vi "DAQ_main.vi"   [LabVIEW 2015]
uses:
  CONTROLS/Q_main_element.ctl
  CONTROLS/Q_DAQ_element.ctl
  <vilib>/DAQmx/write.llb/DAQmx Write (Digital Bool 1Line 1Point).vi
  <vilib>/DAQmx/read.llb/DAQmx Read (Digital Bool 1Line 1Point).vi
  <vilib>/DAQmx/read.llb/DAQmx Read (Counter U32 1Chan 1Samp).vi
  GLOBAL/Global_DAQ.vi
  GLOBAL/Global_ABORT.vi
  GLOBAL/Global_MAIN.vi
  <vilib>/DAQmx/create/channels.llb/DAQmx Create Channel (DO-Digital Output).vi
  <vilib>/DAQmx/miscellaneous.llb/DAQmx Fill In Error Info.vi
  <vilib>/DAQmx/create/channels.llb/DAQmx Create Channel (DI-Digital Input).vi
  <vilib>/DAQmx/create/channels.llb/DAQmx Create Channel (CI-Count Edges).vi
types:
  T1 = cluster{"Analogic input":tag, "size(s)":i32, " waveform":waveform(dbl)}[]
  T2 = cluster{"AOTF trigger task":refnum<k21>, "counter task":refnum<k21>}
  T3 = typedef "Q_DAQ_element.ctl" = cluster{"variant":variant, "Instruction":enum16{"DAQ_idle", "DAQ_initialize", "DAQ_error", "DAQ_security_stop", "DAQ_init_single_scan", "DAQ_single_scan", "DAQ_init_merFISH", "DAQ_scan_merFISH", "DAQ_photobleaching_merFISH", "DAQ_close_merFISH", "DAQ_stop"}}
  T4 = typedef "Q_main_element.ctl" = cluster{"variant":variant, "Instruction":enum16{"Main_idle", "Main_initialize", "Main_initialize_TDMS", "Main_initialize_Queue", "Main_error", "Main_DAQ_initialization_results", "Main_ASI_initialization_results", "Main_Piezo_initialization_results", "Main_Valve_initialization_results", "Main_Pump_initialization_results", "Main_CAMERA_initialization_results", "Main_FPGA_initialization_results", "Main_DAQ_error", "Main_ASI_error", "Main_Piezo_error", "Main_CAMERA_error", "Main_Valve_error", "Main_Pump_error", "Main_FPGA_error", "Main_start_acquiring", "Main_not_acquiring", "Main_acquiring", "Main_stop_acquiring", "Main_change_exposure", "Main_change_z_scan_parameters", "Main_define_ROI", "Main_define_mosaic", "Main_read_kinetic_time", "Main_cooler", "Main_read_temperature", "Main_save_XY", "Main_load_XY", "Main_discard_XY", "Main_move_to_XY", "Main_measure_QPD", "Main_autofocus_calibration", "Main_autofocus_initialization", "Main_autofocus_stop", "Main_save_PID", "Main_change_H_valve_position", "Main_two_way_valve", "Main_save_movie", "Main_init_single_scan", "Main_single_scan", "Main_stop_single_scan", "Main_merFISH_illumination_parameters", "Main_merFISH_buffer_probe_list", "Main_merFISH_injections_procedure", "Main_merFISH_save_setpoint", "Main_merFISH_DAPI_parameters", "Main_merFISH_Brightfield_parameters", "Main_merFISH_save_embryo_ROI", "Main_merFISH_init", "Main_merFISH_resume", "Main_merFISH_start_autofocus", "Main_merFISH_open_close_valve_merFISH", "Main_merFISH_open_close_valve_photobleaching", "Main_merFISH_hybridization", "Main_merFISH_move_to_ROI", "Main_merFISH_wait_stabilization", "Main_merFISH_move_to_REF", "Main_merFISH_scan", "Main_merFISH_photobleaching_injection", "Main_merFISH_photobleaching", "Main_merFISH_send_email", "Main_merFISH_close", "Main_STOP"}}
  T5 = enum16{"DAQ_idle", "DAQ_initialize", "DAQ_error", "DAQ_security_stop", "DAQ_init_single_scan", "DAQ_single_scan", "DAQ_init_merFISH", "DAQ_scan_merFISH", "DAQ_photobleaching_merFISH", "DAQ_close_merFISH", "DAQ_stop"}
  T6 = cluster{"Analogic input":tag, "size(s)":i32, " waveform":waveform(dbl)}
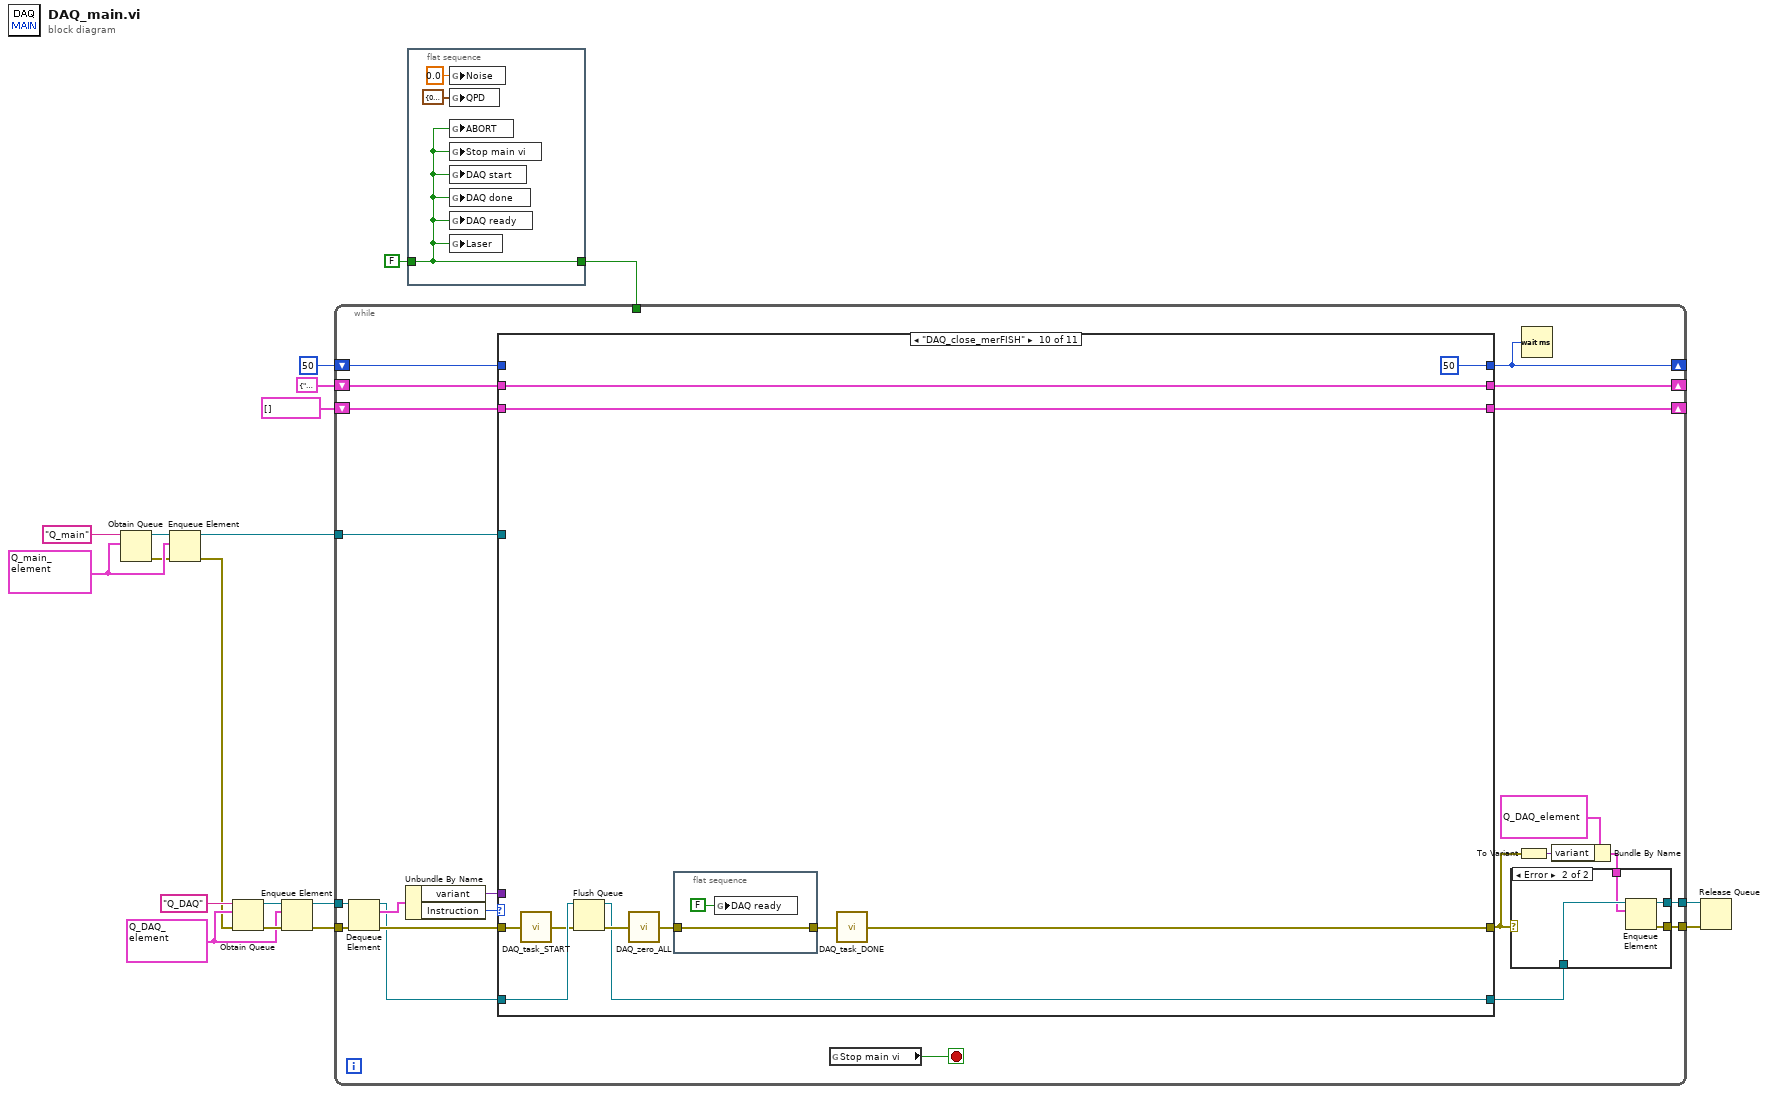
[diagram p0: block diagram]
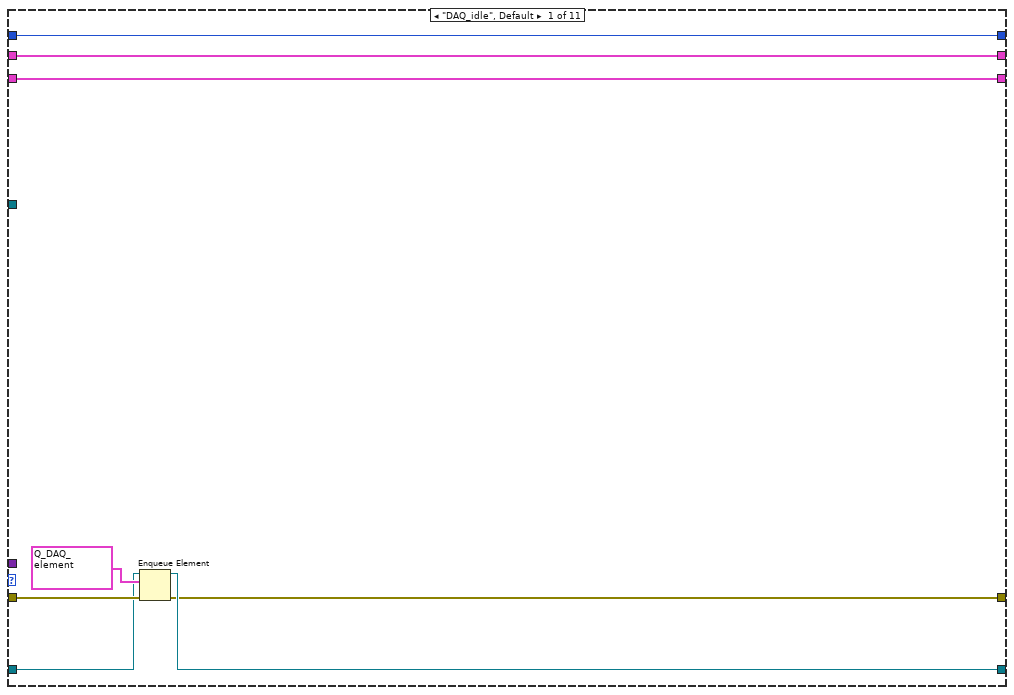
[diagram p3: hidden frame]
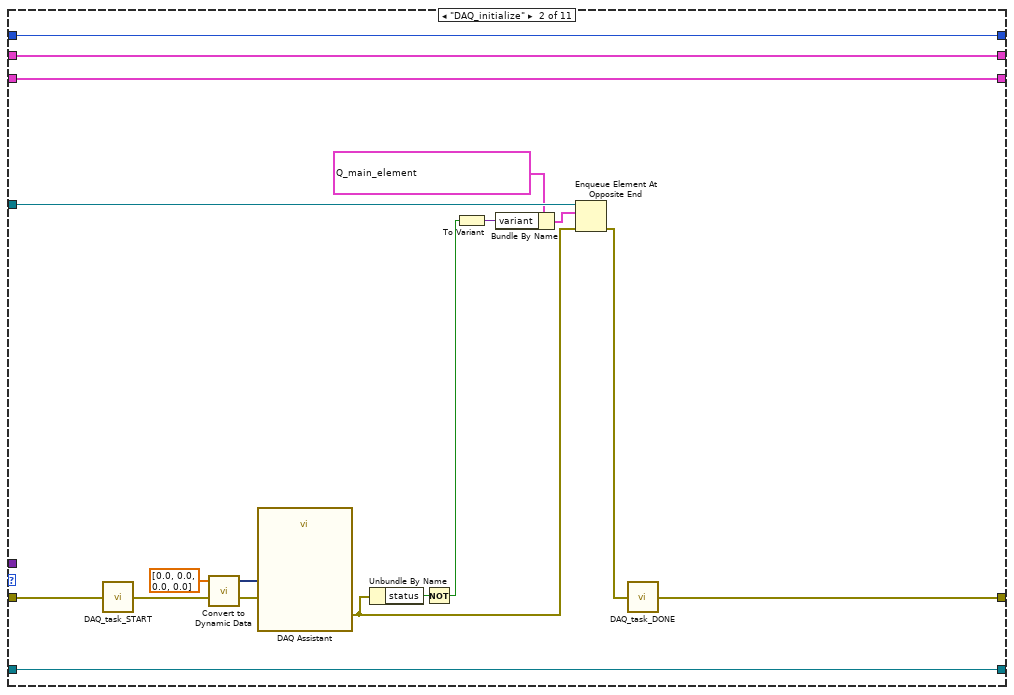
[diagram p4: hidden frame]
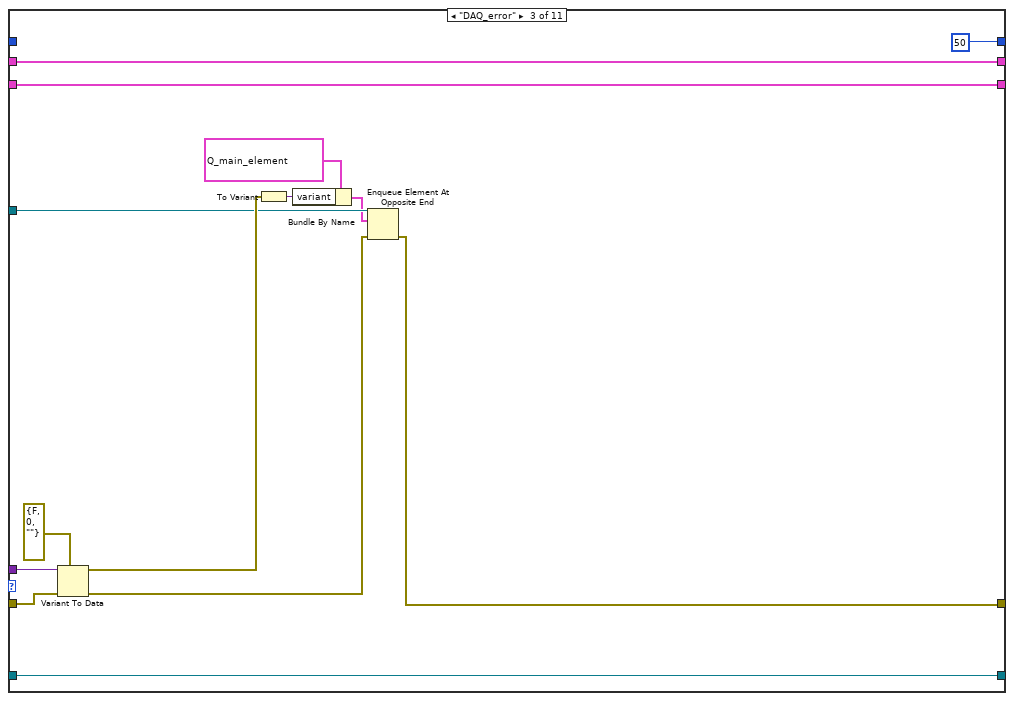
[diagram p5: hidden frame]
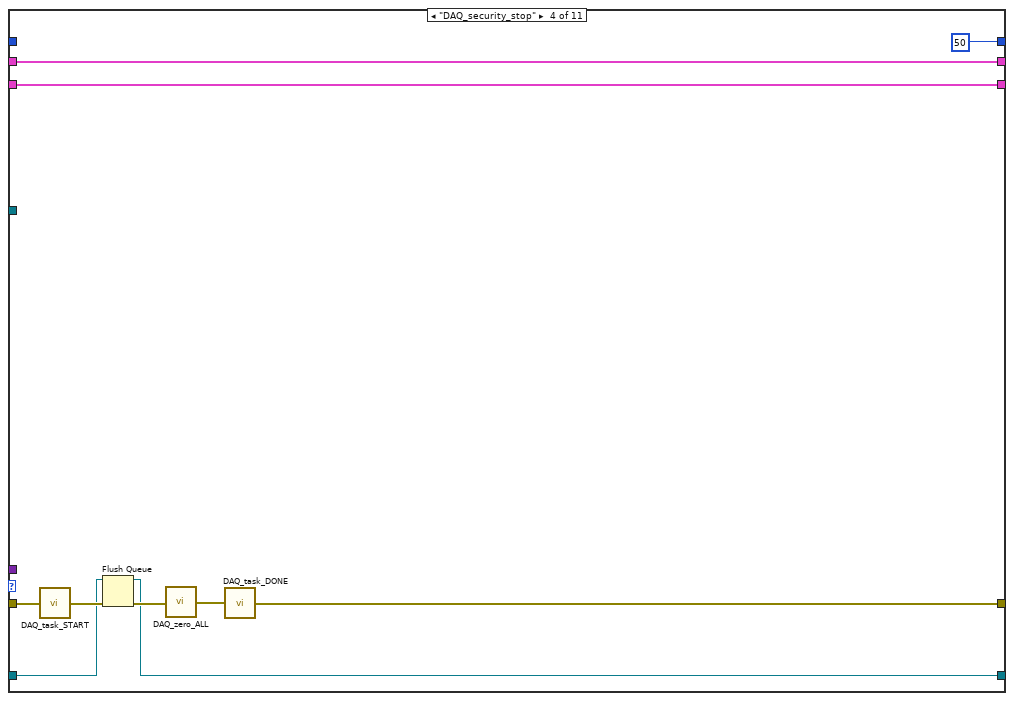
[diagram p6: hidden frame]
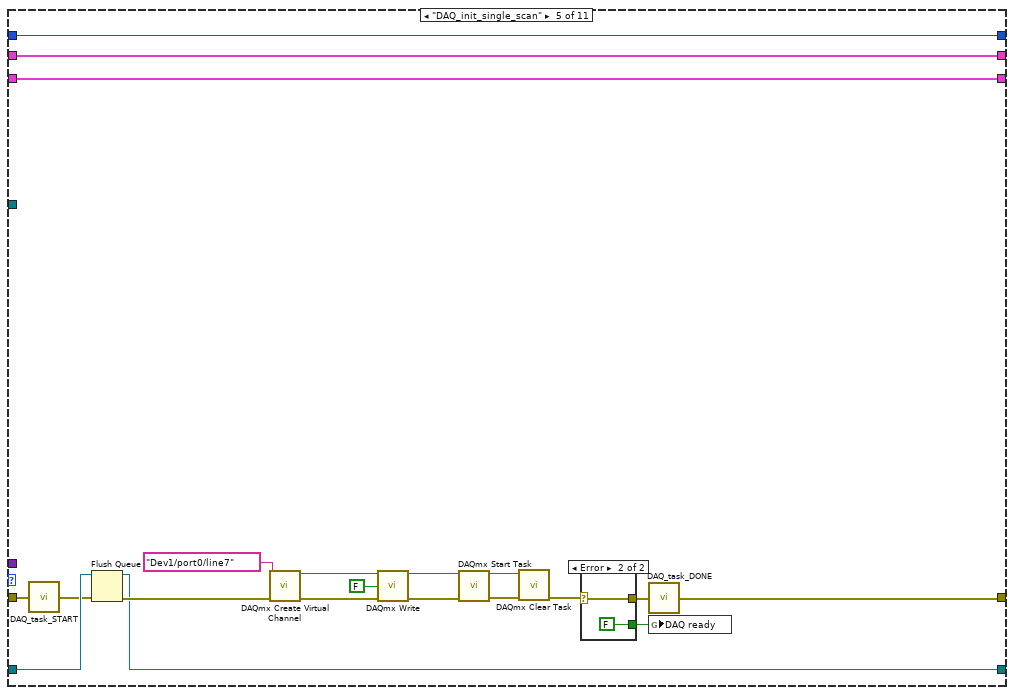
[diagram p7: hidden frame]
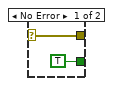
[diagram p8: hidden frame]
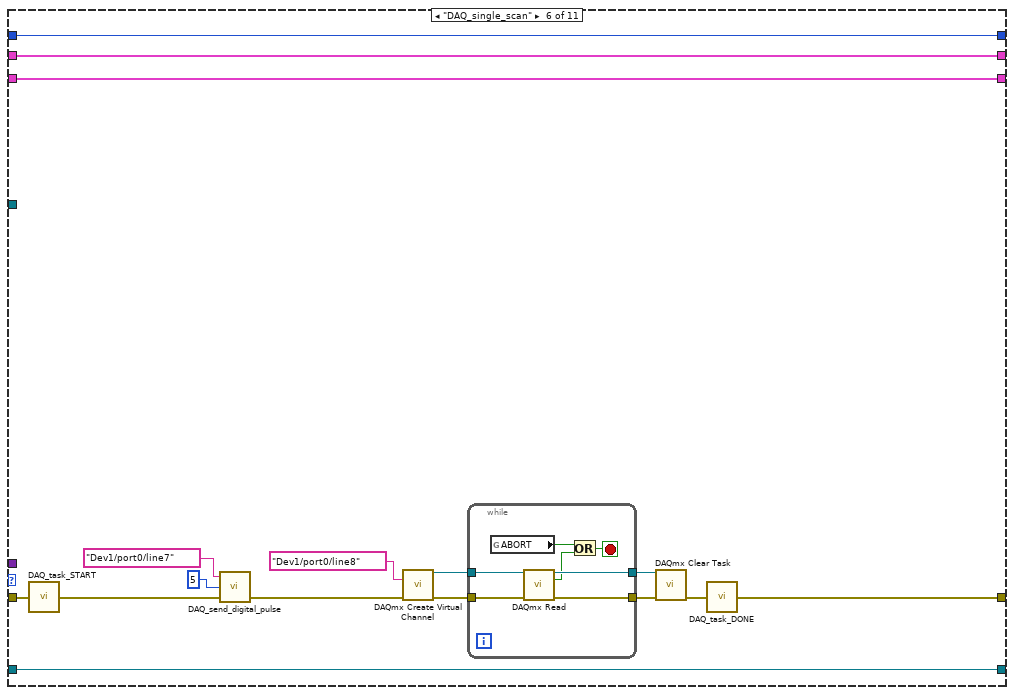
[diagram p9: hidden frame]
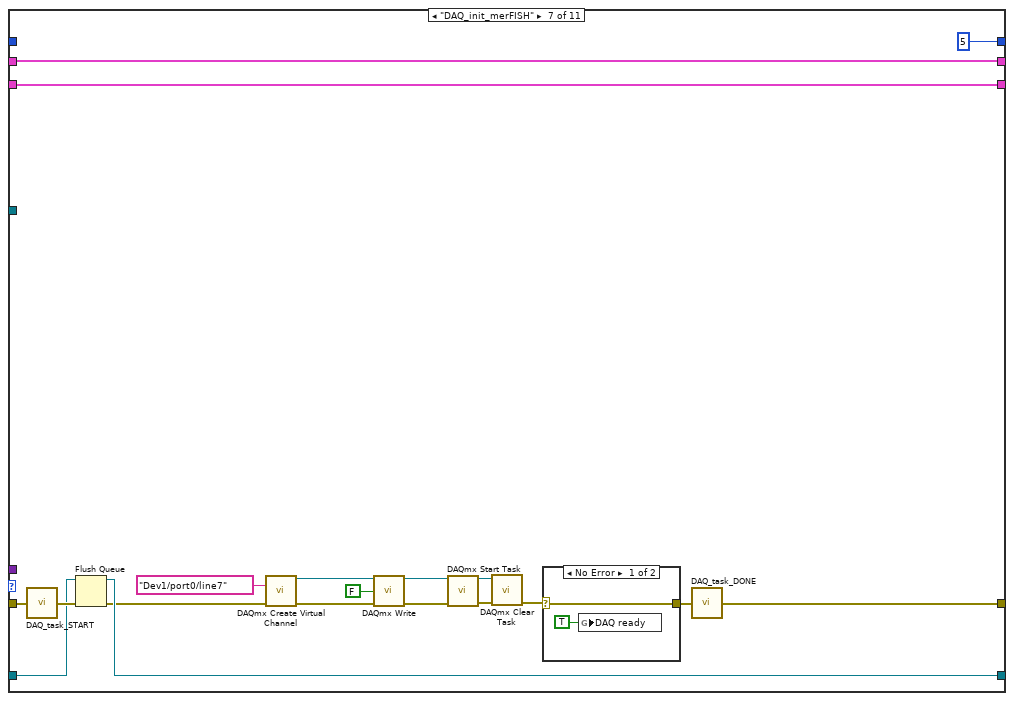
[diagram p10: hidden frame]
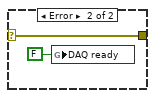
[diagram p11: hidden frame]
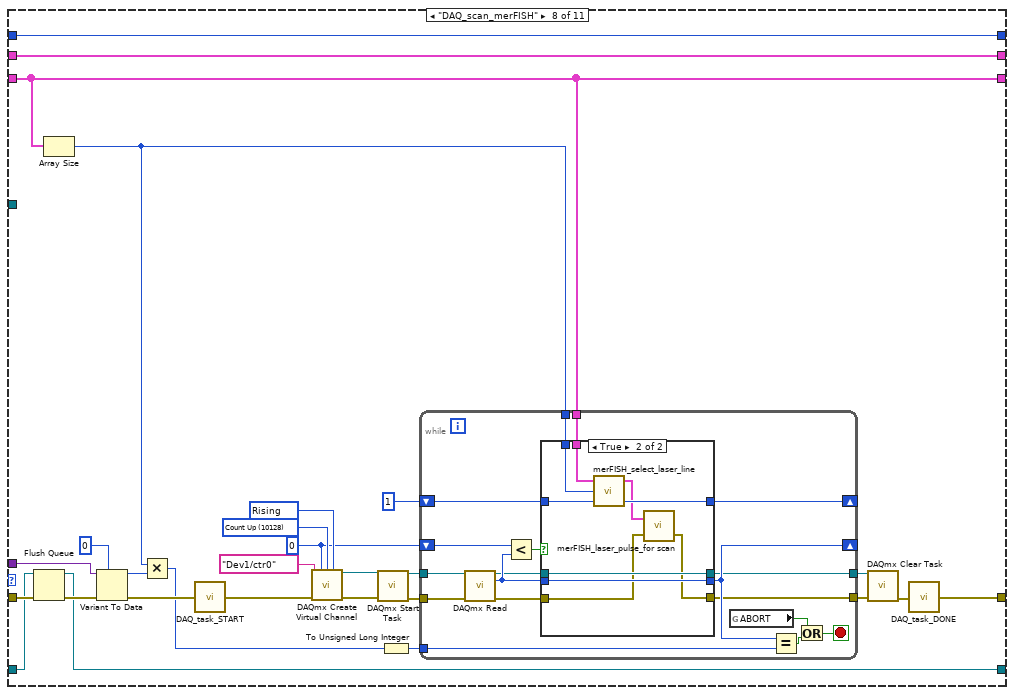
[diagram p12: hidden frame]
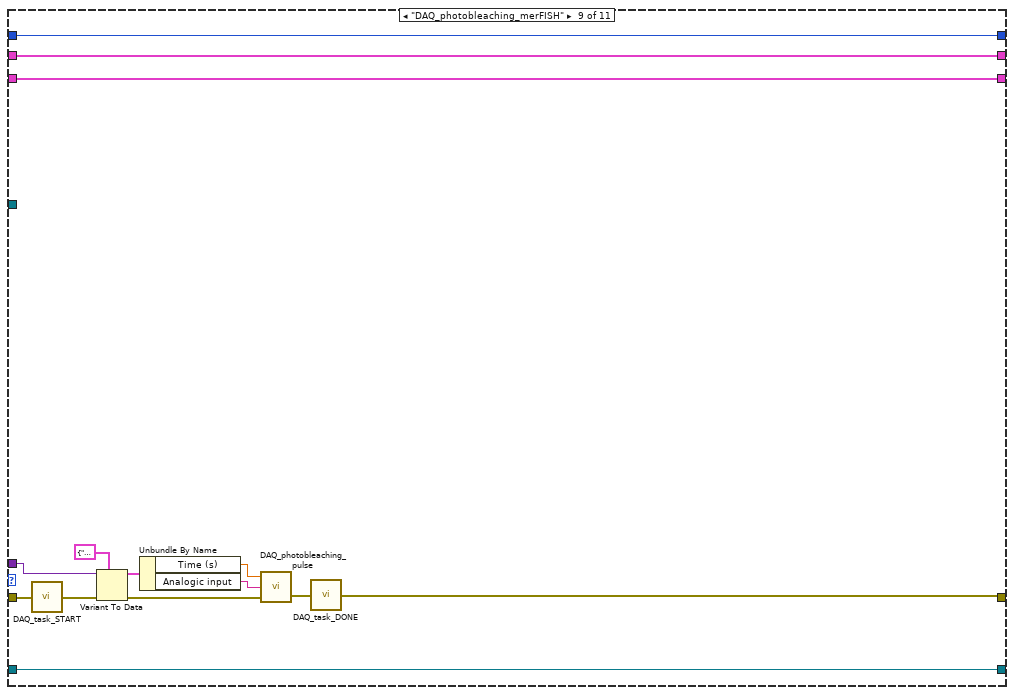
[diagram p14: hidden frame]
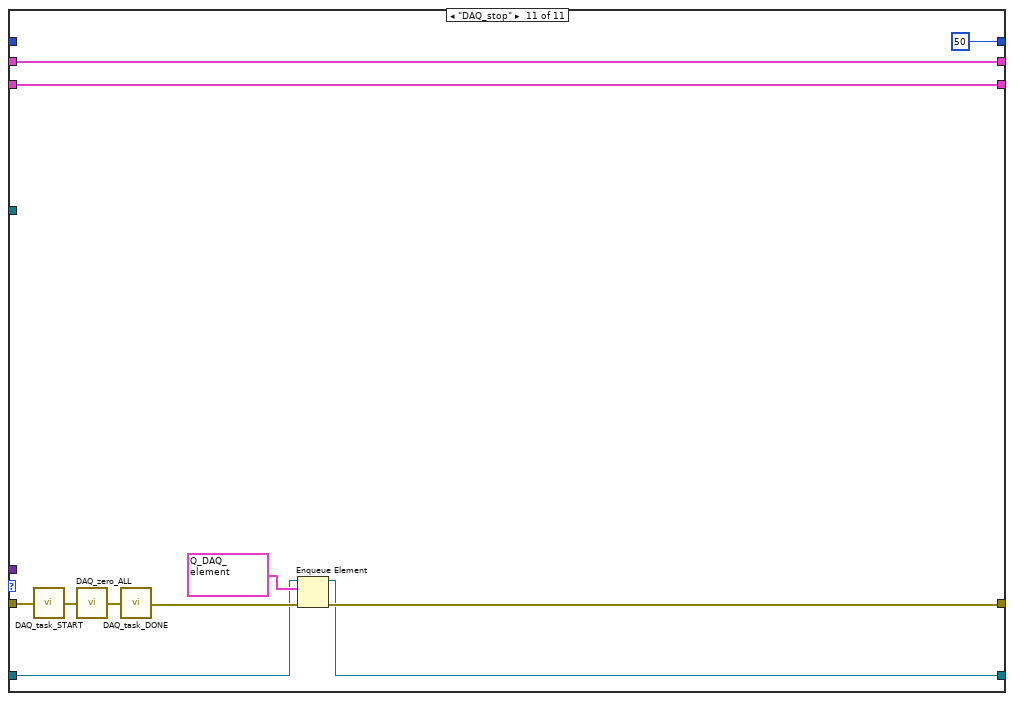
[diagram p15: hidden frame]
diagram:
  w5 = T3 {"variant"=variant, "Instruction"=enum."DAQ_idle"} ("Q_DAQ")
  w12 = T4 {"variant"=variant, "Instruction"=enum."Main_idle"} ("Q_main_element")
  n1 = Obtain Queue(name (unnamed)="Q_main", element data type=w12) -> (queue out=w10:refnum<queue>, error out=w11:errorcluster)  [unwired: 3 in, 1 out]
  n2 = Enqueue Element(queue=w10, element=w12, error in (no error)=w11) -> (queue out=w8:refnum<queue>, error out=w4:errorcluster)  [unwired: 1 in, 1 out]
  n3 = Obtain Queue(name (unnamed)="Q_DAQ", element data type=w5, error in (no error)=w4) -> (queue out=w18:refnum<queue>, error out=w17:errorcluster)  [unwired: 2 in, 1 out]
  n4 = Enqueue Element(queue=w18, element=w5, error in (no error)=w17) -> (queue out=w16:refnum<queue>, error out=w15:errorcluster)  [unwired: 1 in, 1 out]
  n5 = while {
    tunnel: w16 -> [w40]
    tunnel: w15 -> [w39]
    tunnel: [w36] -> w14
    tunnel: [w35] -> w13
    tunnel: w8 -> [w34]
    tunnel: w6 -> [_]
    shift-right: [w27] -> _
    shift-left: T2 {"AOTF trigger task"="", "counter task"=""} ("output cluster") -> [w28]
    shift-right: [w24] -> _
    shift-left: u32 50 ("milliseconds to wait") -> [w25]
    shift-right: [w23] -> _
    shift-left: T1 [] -> [w22]
    stop <- w41 stop-if-true
    n6 = Dequeue Element(queue=w40, error in (no error)=w39) -> (queue out=w21:refnum<queue>, element=w38:T3, error out=w37:errorcluster)  [unwired: 1 in, 1 out]
    n7 = Unbundle By Name(w38) -> ("variant"=w33:variant, "Instruction"=w26:T5)
    n8 = case shown="\"DAQ_close_merFISH\"" w26 {
      tunnel: w37 -> [w52 w57 w85 w96 w99 w133 w158 w192 w237 w245 w262]
      tunnel: [w48 w61 w76 w93 w97 w132 w162 w171 w239 w242 w256] -> w29
      tunnel: w34 -> [_ w70 w80 _ _ _ _ _ _ _ _]
      tunnel: w33 -> [_ _ w86 _ _ _ _ w177 w236 _ _]
      tunnel: w21 -> [w50 w58 w73 w94 w101 w131 w156 w191 w226 w248 w255]
      tunnel: w28 -> [w55 w63 w77 w92 w116 w136 w161 w193 w238 w250 w263]
      tunnel: [w55 w63 w77 w92 w116 w136 w161 w193 w238 w250 w263] -> w27
      tunnel: w25 -> [w54 w60 _ _ w115 w135 _ w194 w228 _ _]
      tunnel: [w54 w60 u32 50 ("milliseconds to wait") u32 50 ("milliseconds to wait") w115 w135 u32 5 ("milliseconds to wait") w194 w228 u32 50 ("milliseconds to wait") u32 50 ("milliseconds to wait")] -> w24
      tunnel: [w53 w59 w74 w88 w114 w134 w144 w181 w227 w246 w259] -> w23
      tunnel: w22 -> [w53 w59 w74 w88 w114 w134 w144 w181 w227 w246 w259]
      tunnel: [w49 w58 w73 w87 w100 w131 w155 w167 w226 w241 w254] -> w20
      frame "DAQ_idle", Default {
        n9 = Enqueue Element(queue=w50, element=T3 {"variant"=variant, "Instruction"=enum."DAQ_idle"} ("Q_DAQ"), error in (no error)=w52) -> (queue out=w49:refnum<queue>, error out=w48:errorcluster)  [unwired: 1 in, 1 out]
      }
      frame "DAQ_initialize" {
        n10 = call "DAQ_task_START.vi"("error in"=w57) -> ("error out"=w64:errorcluster)  [unwired: 1 in]
        n11 = call "Convert to Dynamic Data"("Array"=dbl[] [0.0, 0.0, 0.0, 0.0]) -> ("Dynamic Data Type"=w72:dynamicdata)  [unwired: 3 in]
        n12 = call "DAQ Assistant"("data"=w72, "error in"=w64) -> ("error out"=w62:errorcluster)  [unwired: 16 in, 1 out]
        n13 = Unbundle By Name(w62) -> ("status"=w66:bool)
        n14 = Not(x=w66) -> (.not. x?=w65:bool)
        n15 = To Variant(anything=w65) -> (Variant=w68:variant)
        n16 = Bundle By Name(cluster=T4 {"variant"=variant, "Instruction"=enum."Main_DAQ_initialization_results"} ("element"), "variant"=w68) -> (w67:T4)
        n17 = Enqueue Element At Opposite End(queue=w70, element=w67, error in (no error)=w62) -> (error out=w56:errorcluster)  [unwired: 1 in, 2 out]
        n18 = call "DAQ_task_DONE.vi"("error in"=w56) -> ("error out"=w61:errorcluster)
      }
      frame "DAQ_error" {
        n19 = Variant To Data(error in=w85, type=errorcluster {"status"=FALSE, "code"=0, "source"=""} ("error out"), Variant=w86) -> (data=w81:errorcluster, error out=w79:errorcluster)
        n20 = To Variant(anything=w81) -> (Variant=w82:variant)
        n21 = Bundle By Name(cluster=T4 {"variant"=variant, "Instruction"=enum."Main_DAQ_error"} ("Q_main_element"), "variant"=w82) -> (w78:T4)
        n22 = Enqueue Element At Opposite End(queue=w80, element=w78, error in (no error)=w79) -> (error out=w76:errorcluster)  [unwired: 1 in, 2 out]
      }
      frame "DAQ_security_stop" {
        n23 = call "DAQ_task_START.vi"("error in"=w96) -> ("error out"=w95:errorcluster)  [unwired: 1 in]
        n24 = Flush Queue(queue=w94, error in (no error)=w95) -> (queue out=w87:refnum<queue>, error out=w91:errorcluster)  [unwired: 1 out]
        n25 = call "DAQ_zero_ALL.vi"("error in"=w91) -> ("error out"=w90:errorcluster)
        n26 = call "DAQ_task_DONE.vi"("error in"=w90) -> ("error out"=w93:errorcluster)
      }
      frame "DAQ_init_single_scan" {
        n27 = call "DAQ_task_START.vi"("error in"=w99) -> ("error out"=w98:errorcluster)  [unwired: 1 in]
        n28 = Flush Queue(queue=w101, error in (no error)=w98) -> (queue out=w100:refnum<queue>, error out=w104:errorcluster)  [unwired: 1 out]
        n29 = call-poly <vilib>:"DAQmx Create Virtual Channel.vi"("lines"=tag "Dev1/port0/line7", "error in"=w104) -> ("task out"=w106:refnum<k21>, "error out"=w107:errorcluster)  [unwired: 12 in]
        n30 = call-poly <vilib>:"DAQmx Write.vi"("task/channels in"=w106, "data"=FALSE, "error in"=w107) -> ("task out"=w109:refnum<k21>, "error out"=w110:errorcluster)  [unwired: 10 in, 1 out]
        n31 = call <vilib>:"DAQmx Start Task.vi"("task/channels in"=w109, "error in"=w110) -> ("task out"=w111:refnum<k21>, "error out"=w112:errorcluster)  [unwired: 12 in]
        n32 = call <vilib>:"DAQmx Clear Task.vi"("task in"=w111, "error in"=w112) -> ("error out"=w113:errorcluster)  [unwired: 13 in]
        n33 = case shown="Error" w113 {
          selector: w113 -> [w118 w120]
          tunnel: [w118 w120] -> w102
          tunnel: [TRUE ("DAQ ready") FALSE ("DAQ ready")] -> w103
          frame No Error {
          }
          frame Error {
          }
        }
        n34 = call "DAQ_task_DONE.vi"("error in"=w102) -> ("error out"=w97:errorcluster)
        n35 = global write "Global_DAQ.vi" "DAQ ready"(w103) -> ()
      }
      frame "DAQ_single_scan" {
        n36 = call "DAQ_task_START.vi"("error in"=w133) -> ("error out"=w122:errorcluster)  [unwired: 1 in]
        n37 = call "DAQ_send_digital_pulse.vi"("error in"=w122, "Pulse length (ms)"=u32 5, "Digital input"=tag "Dev1/port0/line7") -> ("error out"=w125:errorcluster)  [unwired: 2 in]
        n38 = call-poly <vilib>:"DAQmx Create Virtual Channel.vi"("lines"=tag "Dev1/port0/line8", "error in"=w125) -> ("task out"=w128:refnum<k21>, "error out"=w127:errorcluster)  [unwired: 12 in]
        n39 = while {
          tunnel: w127 -> [w143]
          tunnel: w128 -> [w142]
          tunnel: [w141] -> w129
          tunnel: [w140] -> w130
          stop <- w139 stop-if-true
          n40 = global read "Global_ABORT.vi" "ABORT"() -> (w137:bool)
          n41 = call-poly <vilib>:"DAQmx Read.vi"("task/channels in"=w142, "error in"=w143) -> ("task out"=w141:refnum<k21>, "data"=w138:bool, "error out"=w140:errorcluster)  [unwired: 11 in]
          n42 = Or(x=w137, y=w138) -> (x .or. y?=w139:bool)
        }
        n43 = call <vilib>:"DAQmx Clear Task.vi"("task in"=w129, "error in"=w130) -> ("error out"=w121:errorcluster)  [unwired: 13 in]
        n44 = call "DAQ_task_DONE.vi"("error in"=w121) -> ("error out"=w132:errorcluster)
      }
      frame "DAQ_init_merFISH" {
        n45 = call "DAQ_task_START.vi"("error in"=w158) -> ("error out"=w157:errorcluster)  [unwired: 1 in]
        n46 = Flush Queue(queue=w156, error in (no error)=w157) -> (queue out=w155:refnum<queue>, error out=w146:errorcluster)  [unwired: 1 out]
        n47 = call-poly <vilib>:"DAQmx Create Virtual Channel.vi"("lines"=tag "Dev1/port0/line7", "error in"=w146) -> ("task out"=w148:refnum<k21>, "error out"=w149:errorcluster)  [unwired: 12 in]
        n48 = call-poly <vilib>:"DAQmx Write.vi"("task/channels in"=w148, "data"=FALSE, "error in"=w149) -> ("task out"=w151:refnum<k21>, "error out"=w152:errorcluster)  [unwired: 10 in, 1 out]
        n49 = call <vilib>:"DAQmx Start Task.vi"("task/channels in"=w151, "error in"=w152) -> ("task out"=w153:refnum<k21>, "error out"=w154:errorcluster)  [unwired: 12 in]
        n50 = call <vilib>:"DAQmx Clear Task.vi"("task in"=w153, "error in"=w154) -> ("error out"=w145:errorcluster)  [unwired: 13 in]
        n51 = case shown="No Error" w145 {
          selector: w145 -> [w164 w166]
          tunnel: [w164 w166] -> w160
          frame No Error {
            n52 = global write "Global_DAQ.vi" "DAQ ready"(TRUE ("DAQ ready")) -> ()
          }
          frame Error {
            n53 = global write "Global_DAQ.vi" "DAQ ready"(FALSE ("DAQ ready")) -> ()
          }
        }
        n54 = call "DAQ_task_DONE.vi"("error in"=w160) -> ("error out"=w162:errorcluster)
      }
      frame "DAQ_scan_merFISH" {
        w188 = 10280 items=["Rising"=10280, "Falling"=10171] ("edge")
        w189 = 10128 items=["Count Up"=10128, "Count Down"=10124, "Externally Controlled"=10326] ("count direction")
        w182 = u32 0 ("initial count")
        n55 = Flush Queue(queue=w191, error in (no error)=w192) -> (queue out=w167:refnum<queue>, error out=w179:errorcluster)  [unwired: 1 out]
        n56 = Array Size(array=w181) -> (size(s)=w174:i32)
        n57 = Variant To Data(error in=w179, type=0 ("Total # z steps"), Variant=w177) -> (data=w175:i32, error out=w178:errorcluster)
        n58 = Multiply(x=w174, y=w175) -> (x*y=w173:i32)
        n59 = call "DAQ_task_START.vi"("error in"=w178) -> ("error out"=w190:errorcluster)  [unwired: 1 in]
        n60 = call-poly <vilib>:"DAQmx Create Virtual Channel.vi"("initial count"=w182, "count direction"=w189, "edge"=w188, "counter"=tag "Dev1/ctr0", "error in"=w190) -> ("task out"=w186:refnum<k21>, "error out"=w185:errorcluster)  [unwired: 9 in]
        n61 = call <vilib>:"DAQmx Start Task.vi"("task/channels in"=w186, "error in"=w185) -> ("task out"=w183:refnum<k21>, "error out"=w184:errorcluster)  [unwired: 12 in]
        n62 = To Unsigned Long Integer(number=w173) -> (unsigned 32bit integer=w172:u32)
        n63 = while {
          tunnel: w184 -> [w211]
          tunnel: w183 -> [w212]
          shift-right: [w202] -> _
          shift-left: w182 -> [w210]
          tunnel: w174 -> [w205]
          tunnel: w181 -> [w206]
          shift-right: [w203] -> _
          shift-left: 1 ("initial count") -> [w204]
          tunnel: w172 -> [w201]
          tunnel: [w198] -> w169
          tunnel: [w199] -> w170
          stop <- w195 stop-if-true
          n64 = call-poly <vilib>:"DAQmx Read.vi"("task/channels in"=w212, "error in"=w211) -> ("task out"=w200:refnum<k21>, "data"=w207:u32, "error out"=w208:errorcluster)  [unwired: 11 in]
          n65 = Less?(x=w210, y=w207) -> (x < y?=w209:bool)
          n66 = case shown="True" w209 {
            tunnel: w208 -> [w214 w218]
            tunnel: w207 -> [w215 w225]
            tunnel: [w215 w225] -> w202
            tunnel: w206 -> [_ w224]
            tunnel: w205 -> [_ w223]
            tunnel: w204 -> [w216 w222]
            tunnel: [w216 w221] -> w203
            tunnel: [w214 w217] -> w198
            tunnel: w200 -> [w213 w219]
            tunnel: [w213 w219] -> w199
            frame False {
            }
            frame True {
              n67 = call "merFISH_select_laser_line.vi"("Laser line"=w222, "Total number of lines"=w223, "Laser array"=w224) -> ("Next laser line"=w221:i32, "excitation cluster"=w220:T6)  [unwired: 1 in]
              n68 = call "merFISH_laser_pulse_for scan.vi"("error in"=w218, "excitation cluster"=w220) -> ("error out"=w217:errorcluster)  [unwired: 1 in]
            }
          }
          n69 = global read "Global_ABORT.vi" "ABORT"() -> (w196:bool)
          n70 = Equal?(x=w202, y=w201) -> (x = y?=w197:bool)
          n71 = Or(x=w196, y=w197) -> (x .or. y?=w195:bool)
        }
        n72 = call <vilib>:"DAQmx Clear Task.vi"("task in"=w170, "error in"=w169) -> ("error out"=w168:errorcluster)  [unwired: 13 in]
        n73 = call "DAQ_task_DONE.vi"("error in"=w168) -> ("error out"=w171:errorcluster)
      }
      frame "DAQ_photobleaching_merFISH" {
        n74 = call "DAQ_task_START.vi"("error in"=w237) -> ("error out"=w235:errorcluster)  [unwired: 1 in]
        n75 = Variant To Data(error in=w235, type=cluster{"Analogic input":tag, "Time (s)":dbl} {"Analogic input"="", "Time (s)"=0.0} ("output cluster"), Variant=w236) -> (data=w233:cluster{"Analogic input":tag, "Time (s)":dbl}, error out=w232:errorcluster)
        n76 = Unbundle By Name(w233) -> ("Time (s)"=w230:dbl, "Analogic input"=w231:tag)
        n77 = call "DAQ_photobleaching_pulse.vi"("error in"=w232, "physical channels"=w231, "Pulse length Ton (s)"=w230) -> ("error out"=w229:errorcluster)  [unwired: 1 in]
        n78 = call "DAQ_task_DONE.vi"("error in"=w229) -> ("error out"=w239:errorcluster)
      }
      frame "DAQ_close_merFISH" {
        n79 = call "DAQ_task_START.vi"("error in"=w245) -> ("error out"=w244:errorcluster)  [unwired: 1 in]
        n80 = Flush Queue(queue=w248, error in (no error)=w244) -> (queue out=w241:refnum<queue>, error out=w243:errorcluster)  [unwired: 1 out]
        n81 = call "DAQ_zero_ALL.vi"("error in"=w243) -> ("error out"=w240:errorcluster)
        n82 = flat-sequence {
          tunnel: [w251] -> w247
          tunnel: w240 -> [w251]
          frame #0 {
            n83 = global write "Global_DAQ.vi" "DAQ ready"(FALSE ("DAQ ready")) -> ()
          }
        }
        n84 = call "DAQ_task_DONE.vi"("error in"=w247) -> ("error out"=w242:errorcluster)
      }
      frame "DAQ_stop" {
        n85 = call "DAQ_task_START.vi"("error in"=w262) -> ("error out"=w253:errorcluster)  [unwired: 1 in]
        n86 = call "DAQ_zero_ALL.vi"("error in"=w253) -> ("error out"=w260:errorcluster)
        n87 = call "DAQ_task_DONE.vi"("error in"=w260) -> ("error out"=w257:errorcluster)
        n88 = Enqueue Element(queue=w255, element=T3 {"variant"=variant, "Instruction"=enum."DAQ_idle"} ("Q_DAQ"), error in (no error)=w257) -> (queue out=w254:refnum<queue>, error out=w256:errorcluster)  [unwired: 1 in, 1 out]
      }
    }
    n89 = global read "Global_MAIN.vi" "Stop main vi"() -> (w41:bool)
    n90 = To Variant(anything=w29) -> (Variant=w30:variant)
    n91 = Wait (ms)(milliseconds to wait=w24) -> ()  [unwired: 1 out]
    n92 = Bundle By Name(cluster=T3 {"variant"=variant, "Instruction"=enum."DAQ_error"} ("Q_DAQ"), "variant"=w30) -> (w31:T3)
    n93 = case shown="Error" w29 {
      selector: w29 -> [w43 _]
      tunnel: [w42 w46] -> w36
      tunnel: [w43 w47] -> w35
      tunnel: w20 -> [w42 w45]
      tunnel: w31 -> [_ w44]
      frame No Error {
      }
      frame Error {
        n94 = Enqueue Element(queue=w45, element=w44) -> (queue out=w46:refnum<queue>, error out=w47:errorcluster)  [unwired: 2 in, 1 out]
      }
    }
  }
  n95 = flat-sequence {
    tunnel: FALSE ("Stop main vi") -> [w266]
    tunnel: [w266] -> w6
    frame #0 {
      n96 = global write "Global_DAQ.vi" "Noise"(0.0 ("Noise")) -> ()
      n97 = global write "Global_DAQ.vi" "QPD"(cluster{"X":dbl, "Y":dbl, "intensity":dbl} {"X"=0.0, "Y"=0.0, "intensity"=0.0} ("QPD")) -> ()
      n98 = global write "Global_ABORT.vi" "ABORT"(w266) -> ()
      n99 = global write "Global_MAIN.vi" "Stop main vi"(w266) -> ()
      n100 = global write "Global_DAQ.vi" "DAQ start"(w266) -> ()
      n101 = global write "Global_DAQ.vi" "DAQ done"(w266) -> ()
      n102 = global write "Global_DAQ.vi" "DAQ ready"(w266) -> ()
      n103 = global write "Global_DAQ.vi" "Laser"(w266) -> ()
    }
  }
  n104 = Release Queue(queue=w14, error in (no error)=w13) -> ()  [unwired: 1 in, 3 out]
